vi "niFPGA Dead Zone_m.vi"   [LabVIEW 2017]
doc: "Provides a region of zero output, or a dead zone. <B>output</B> is zero if <B>start of dead zone</B> <= <B>input</B> <= <B>end of dead zone</B>. The data type you wire to <B>input</B> determines the <B>output</B> data type."
uses:
  <vilib>/rvi/Analysis/common/FxpNativeNode/niFpgaFxpNative.xnode
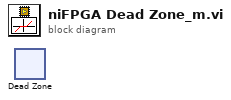
[diagram p0: block diagram]
diagram:
  n1 = xnode "Dead Zone"() -> ()  [unwired: 3 in, 1 out]
